vi "Braise.vi"(8 "error in (no error)":errorcluster, 11 "Microwave in":refnum<class "Microwave.lvclass">) -> (0 "error out":errorcluster, 3 "Microwave out":refnum<class "Microwave.lvclass">)   [LabVIEW 2020, in "Microwave.lvclass"]
uses:
  Microwave.lvclass
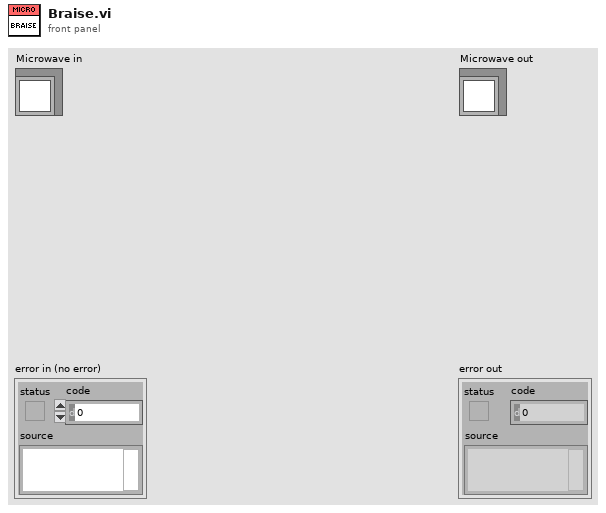
[diagram p1: front panel]
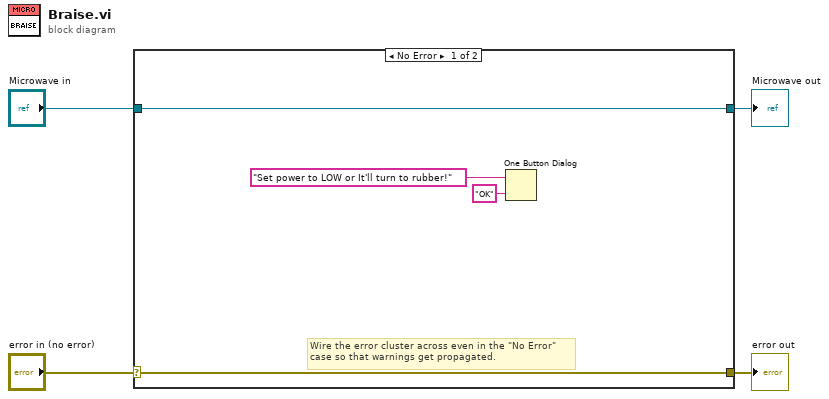
[diagram p0: block diagram]
diagram:
  n1 = case shown="No Error" "error in (no error)" {
    selector: "error in (no error)" -> [w7 w10]
    tunnel: [w7 w10] -> w3
    tunnel: [w8 w9] -> w1
    tunnel: "Microwave in" -> [w8 w9]
    frame No Error {
      # "Wire the error cluster across even in the \"No Error\"\ncase so that warnings get propagated."
      n2 = One Button Dialog(message="Set power to LOW or It'll turn to rubber!", button name ("OK")="OK") -> ()  [unwired: 1 out]
    }
    frame Error {
    }
  }
  "error out" <- w3
  "Microwave out" <- w1
